vi "drawMouseClicks.vi"(8 "error in (no error)":errorcluster, 10 "Current Image in":T1, 11 "mouse click path":string) -> (0 "error out":errorcluster, 3 "Current Image out":T1)   [LabVIEW 2018, in "Image_Diff.lvlib"]
uses:
  Image_Diff.lvlib
  <vilib>/picture/picture.llb/imagedata.ctl
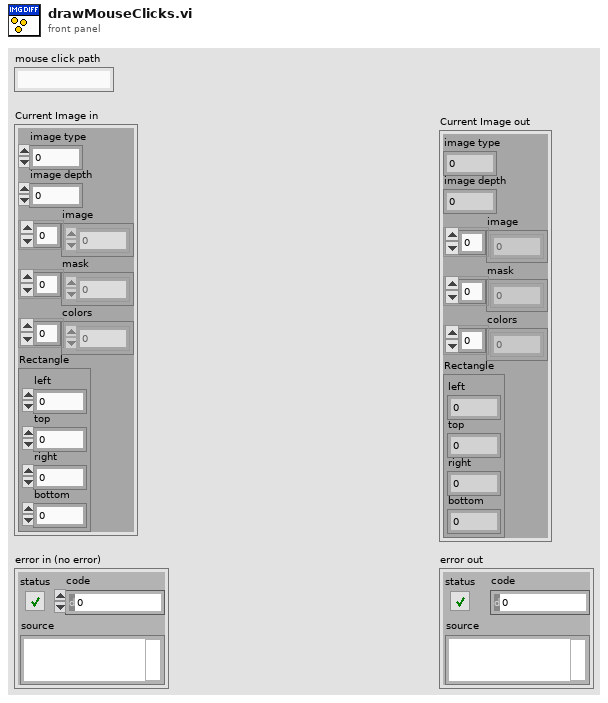
[diagram p1: front panel]
types:
  T1 = typedef "imagedata.ctl" = cluster{"image type":i32, "image depth":i32, "image":u8[], "mask":u8[], "colors":u32[], "Rectangle":cluster{"left":i16, "top":i16, "right":i16, "bottom":i16}}
  T2 = enum16{"User-specified Font", "Application Font", "System Font", "Dialog Font"}
  T3 = cluster{"Font Name:":string, "Size":i16, "Strikeout?":bool, "Italic?":bool, "Underline?":bool, "Outline?":bool, "Shadow?":bool, "Bold?":bool}
  T4 = enum16{"open", "replace", "create", "open or create", "replace or create", "replace or create with confirmation"}
  T5 = cluster{"left":i16, "top":i16, "right":i16, "bottom":i16}
  T6 = cluster{"Width":u16, "Style":enum32{"Solid", "Dash", "Dot", "DashDot", "DashDotDot"}}
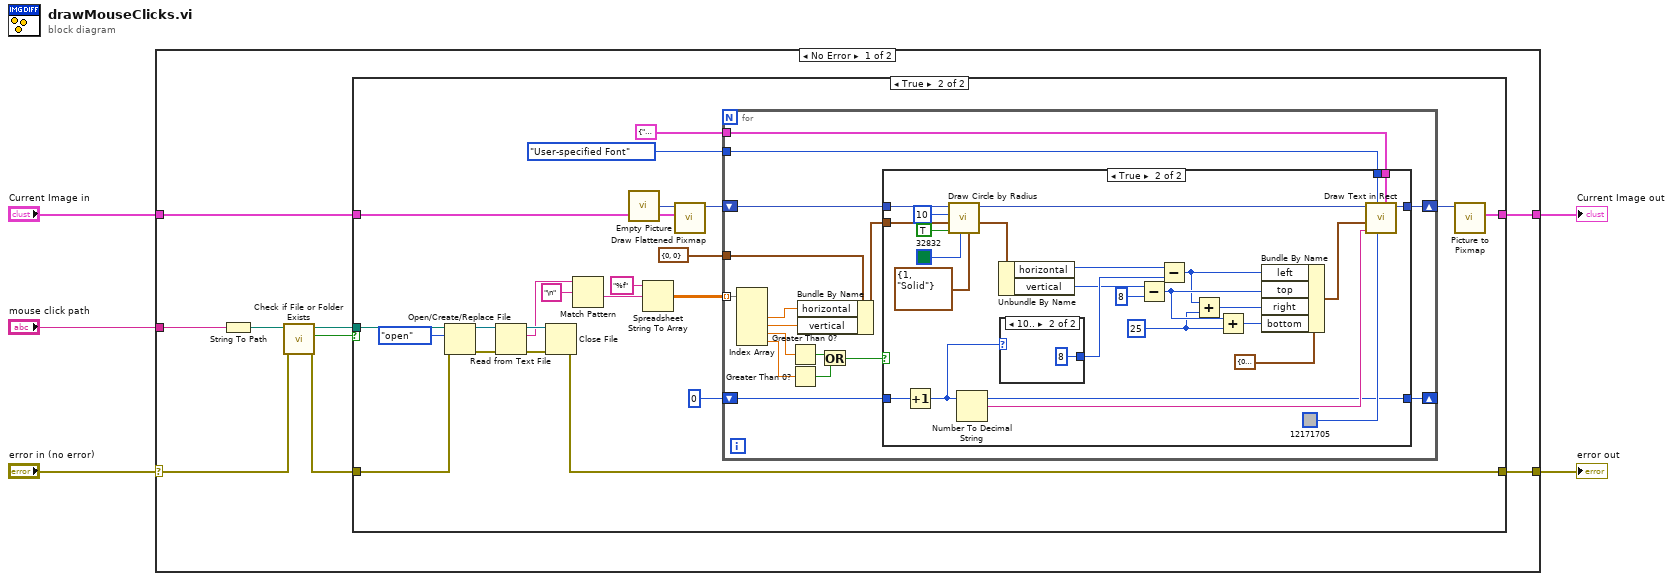
[diagram p0: block diagram]
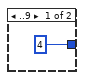
[diagram p4: hidden frame]
diagram:
  n1 = case shown="No Error" "error in (no error)" {
    selector: "error in (no error)" -> [w8 w84]
    tunnel: "mouse click path" -> [w9 _]
    tunnel: "Current Image in" -> [w14 w85]
    tunnel: [w13 w85] -> w3
    tunnel: [w12 w84] -> w2
    frame No Error {
      n2 = String To Path(string=w9) -> (path=w11:path)
      n3 = call <vilib>:"Check if File or Folder Exists.vi"("error in (no error)"=w8, "path"=w11) -> ("error out"=w7:errorcluster, "file or folder exists?"=w6:bool, "dup path"=w10:path)  [unwired: 7 in]
      n4 = case shown="True" w6 {
        tunnel: w14 -> [w16 w28]
        tunnel: [w16 w24] -> w13
        tunnel: [w15 w22] -> w12
        tunnel: w10 -> [_ w21]
        tunnel: w7 -> [w15 w20]
        frame False {
        }
        frame True {
          n5 = Open/Create/Replace File(file path (use dialog)=w21, error in=w20, operation (0:open)=T4."open") -> (refnum out=w36:refnum<file>, error out=w37:errorcluster)  [unwired: 3 in, 1 out]
          n6 = Read from Text File(file (use dialog)=w36, error in=w37) -> (refnum out=w34:refnum<file>, text=w31:string, error out=w35:errorcluster)  [unwired: 2 in, 1 out]
          n7 = Close File(refnum=w34, error in=w35) -> (error out=w22:errorcluster)  [unwired: 1 out]
          n8 = Match Pattern(string=w31, regular expression="\n") -> (after substring=w30:string)  [unwired: 1 in, 3 out]
          n9 = call "Empty Picture"() -> ("empty picture"=w26:picture)
          n10 = Spreadsheet String To Array(format string="%f", spreadsheet string=w30) -> (array=w29:dbl[][])  [unwired: 2 in]
          n11 = call <vilib>:"Draw Flattened Pixmap.vi"("image data"=w28, "picture"=w26) -> ("new picture"=w27:picture)  [unwired: 7 in]
          n12 = for {
            tunnel: w29 -> [w54] mode=indexing
            shift-right: [w49] -> w25
            shift-left: w27 -> [w53]
            tunnel: cluster{"horizontal":i16, "vertical":i16} {"horizontal"=0, "vertical"=0} ("pixel center") -> [w52]
            tunnel: T3 {"Font Name:"="Arial", "Size"=18, "Strikeout?"=FALSE, "Italic?"=FALSE, "Underline?"=FALSE, "Outline?"=FALSE, "Shadow?"=FALSE, "Bold?"=TRUE} ("[user-specified font]") -> [w48]
            tunnel: T2."User-specified Font" ("desired font(Application)") -> [w47]
            shift-right: [w39] -> _
            shift-left: 0 -> [w45]
            n13 = Index Array(array=w54) -> (element #2=w51:dbl, element #3=w50:dbl, element #4=w44:dbl, element #5=w43:dbl)  [unwired: 5 in, 1 out]
            n14 = Greater Than 0?(x=w44) -> (x > 0?=w42:bool)
            n15 = Greater Than 0?(x=w43) -> (x > 0?=w41:bool)
            n16 = Bundle By Name(cluster=w52, "horizontal"=w51, "vertical"=w50) -> (w46:cluster{"horizontal":i16, "vertical":i16})
            n17 = Or(x=w42, y=w41) -> (x .or. y?=w40:bool)
            n18 = case shown="True" w40 {
              tunnel: w53 -> [w56 w81]
              tunnel: [w56 w75] -> w49
              tunnel: w48 -> [_ w73]
              tunnel: w47 -> [_ w72]
              tunnel: w46 -> [_ w59]
              tunnel: w45 -> [w55 w58]
              tunnel: [w55 w57] -> w39
              frame False {
              }
              frame True {
                w63 = i16 25 ("y")
                n19 = Increment(x=w58) -> (x+1=w57:i32)
                n20 = call <vilib>:"Draw Circle by Radius.vi"("pen"=T6 {"Width"=1, "Style"=enum."Solid"}, "color(black)"=u32 32832, "fill?(F)"=TRUE, "pixel center"=w59, "radius"=i16 10, "picture"=w81) -> ("new picture"=w76:picture)  [unwired: 5 in]
                n21 = Number To Decimal String(number=w57) -> (decimal integer string=w71:string)  [unwired: 1 in]
                n22 = Unbundle By Name(w59) -> ("horizontal"=w64:i16, "vertical"=w65:i16)
                n23 = case shown="10.." w57 {
                  tunnel: [i16 4 ("y") i16 8 ("y")] -> w70
                  frame ..9 {
                  }
                  frame 10.. {
                  }
                }
                n24 = Subtract(x=w65, y=i16 8) -> (x-y=w68:i16)
                n25 = Subtract(x=w64, y=w70) -> (x-y=w66:i16)
                n26 = Add(x=w66, y=w63) -> (x+y=w67:i16)
                n27 = Add(x=w68, y=w63) -> (x+y=w69:i16)
                n28 = Bundle By Name(cluster=T5 {"left"=0, "top"=0, "right"=0, "bottom"=0} ("rect"), "left"=w66, "top"=w68, "right"=w67, "bottom"=w69) -> (w60:T5)
                n29 = call <vilib>:"Draw Text in Rect.vi"("[user-specified font]"=w73, "text color(black)"=u32 12171705, "desired font(Application)"=w72, "text"=w71, "rect"=w60, "picture"=w76) -> ("new picture"=w75:picture)  [unwired: 5 in]
              }
            }
          }
          n30 = call <vilib>:"Picture to Pixmap.vi"("picture"=w25) -> ("image data"=w24:T1)  [unwired: 9 in, 1 out]
        }
      }
    }
    frame Error {
    }
  }
  "error out" <- w2
  "Current Image out" <- w3
